vi "CheckCore.vi"(8 "error in (no error)":errorcluster, 9 "# of Refs":i32, 10 "References":refnum<vi>[](array[refnum]), 11 "Blacklist in":refnum<class "Blacklist.lvclass">) -> (0 "error out":errorcluster, 1 "Reject?":bool, 2 "dup References":refnum<vi>[](array[refnum]), 3 "Blacklist out":refnum<class "Blacklist.lvclass">)   [LabVIEW 2014, in "lvbuildsecurity.lvlib" / "Blacklist.lvclass"]
uses:
  Blacklist.lvclass
  Blacklist.lvclass/Blacklist.ctl
  <vilib>/Wiresmith Technology/LabVIEW CLI/CLI Class/CLI.lvclass
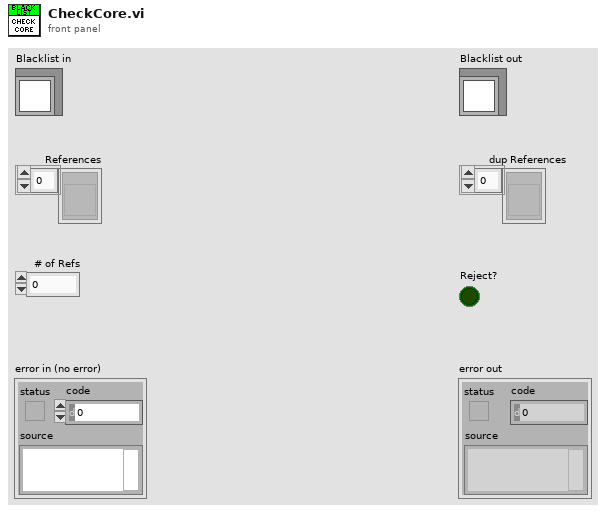
[diagram p1: front panel]
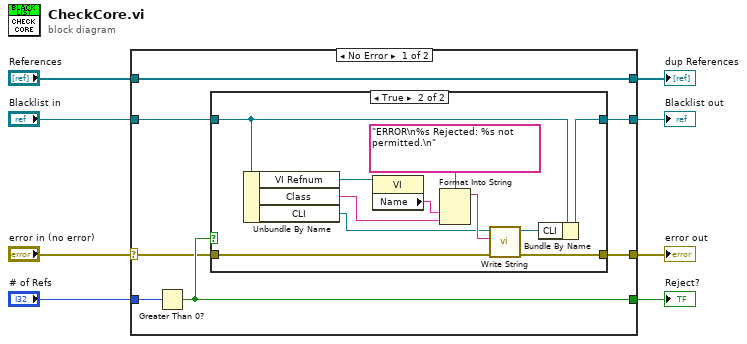
[diagram p0: block diagram]
diagram:
  n1 = case shown="No Error" "error in (no error)" {
    selector: "error in (no error)" -> [w10 w31]
    tunnel: [w9 w31] -> w7
    tunnel: [w12 w30] -> w5
    tunnel: "Blacklist in" -> [w13 w30]
    tunnel: "References" -> [w14 w29]
    tunnel: "# of Refs" -> [w15 _]
    tunnel: [w14 w29] -> w3
    tunnel: [w11 _] -> w2
    frame No Error {
      n2 = Greater Than 0?(x=w15) -> (x > 0?=w11:bool)
      n3 = case shown="True" w11 {
        tunnel: w13 -> [w17 w20]
        tunnel: [w17 w19] -> w12
        tunnel: w10 -> [w16 w22]
        tunnel: [w16 w21] -> w9
        frame False {
        }
        frame True {
          n4 = Unbundle By Name(w20) -> ("VI Refnum"=w28:refnum<vi>, "Class"=w25:string, "CLI"=w23:refnum<class "CLI.lvclass">)
          n5 = property class="VI"(reference=w28) -> ("Name"=w26:string)  [unwired: 1 in, 2 out]
          n6 = Format Into String(format string="ERROR\n%s Rejected: %s not permitted.\n", w26, w25) -> (resulting string=w24:string)  [unwired: 2 in, 1 out]
          n7 = call <vilib>:"Write String.vi"("error in (no error)"=w22, "Text to Write"=w24, "CLI in"=w23) -> ("error out"=w21:errorcluster, "CLI out"=w18:refnum<class "CLI.lvclass">)  [unwired: 7 in]
          n8 = Bundle By Name(cluster=w20, "CLI"=w18) -> (w19:refnum<class "Blacklist.lvclass">)
        }
      }
    }
    frame Error {
    }
  }
  "error out" <- w7
  "Blacklist out" <- w5
  "dup References" <- w3
  "Reject?" <- w2
